vi "SetAtributes.vi"() -> ()   [LabVIEW 2012]
uses:
  <vilib>/Instr/_visa.llb/VISA Configure Serial Port (Instr).vi
panel:
  out "Coef start vasak":string
  out "Coef start parem":string
  in  "Vasak":bool
  out "Konstant vasak":dbl format="%#_4g"
  in  "Raskus vasak":dbl=200.0
  out "Coef OUT vasak":string
  out "Coef IN vasak":string
  in  "Parem":bool
  out "Coef IN parem":string
  out "Coef OUT parem":string
  out "Konstant parem":dbl format="%#_4g"
  in  "Raskus parem":dbl=200.0
  out "parem":dbl
  out "vasak":dbl
  in  "Mitu väärtust":i32=100
  in  "Kalibreeri":bool
  out "Pausi (oote) perioodi vaste":string
  in  "Pausi (oote) periood":string
  out "Salvestusperioodi vaste":string
  in  "Salvestusperiood":string
  out "Max vaste":string
  in  "Max":string
  in  "Pausi (oote) periood":bool
  in  "Salvestusperiood":bool
  in  "Max lävend":bool
  out "Aja vaste":string
  out "Min vaste":string
  in  "Min":string
  in  "Säti min lävend":bool
  in  "stop":bool
  in  "Säti aeg":bool
  in  "Kell":string
  in  "Kuupäev":string
  out "string 4":string
  in  "VISA Refnum in":refnum<visa-resource-name>="COM1"
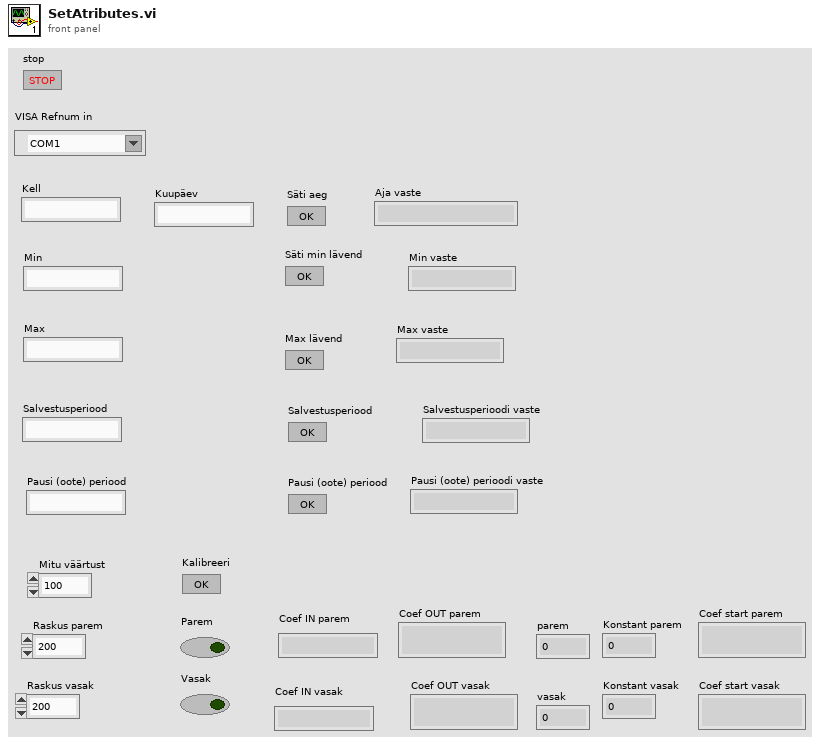
[diagram p1: front panel]
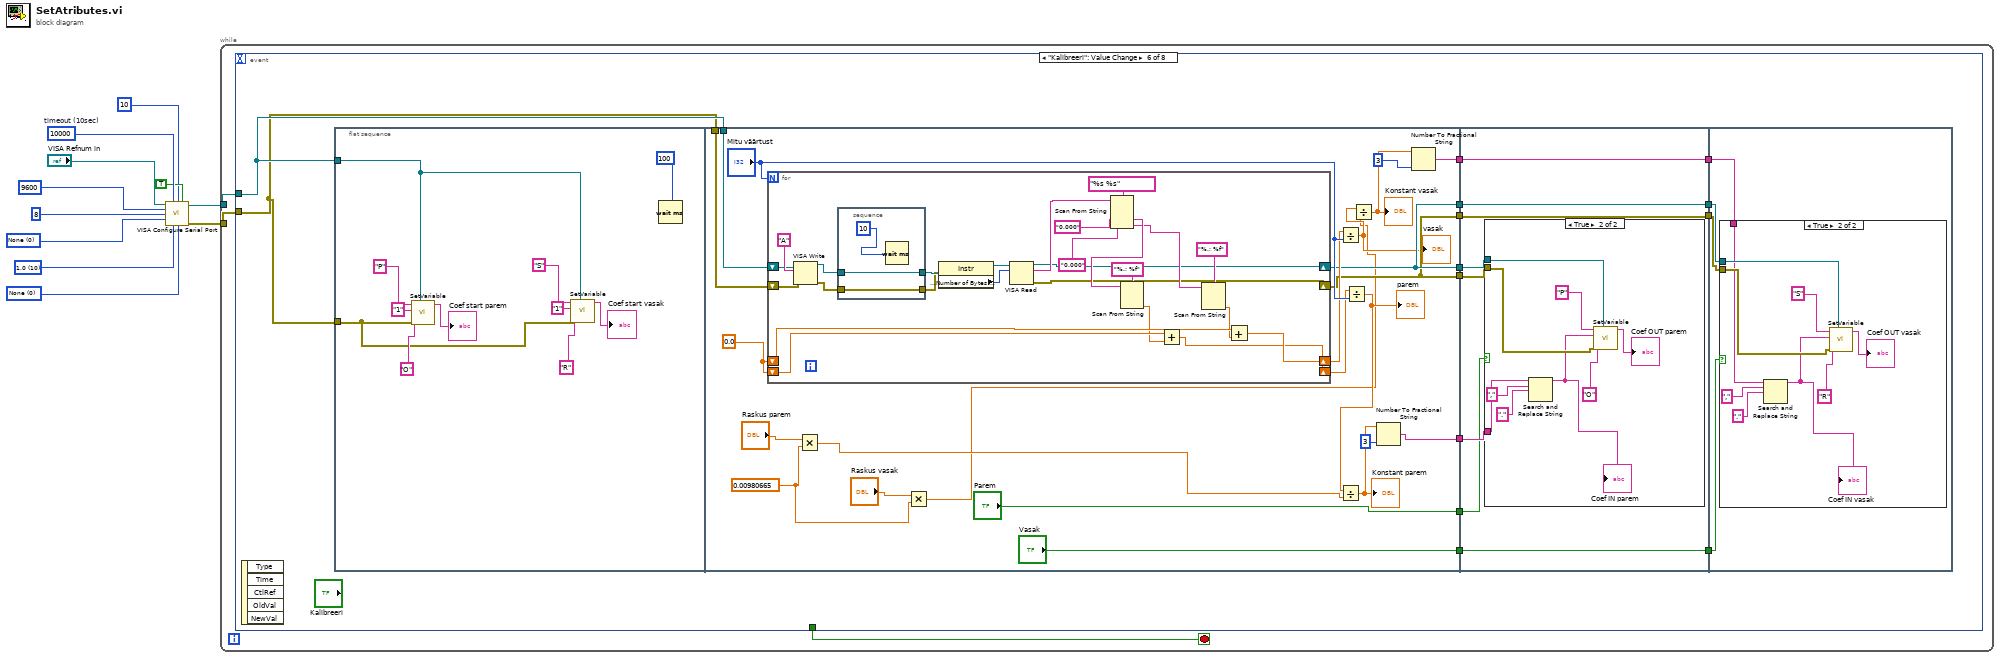
[diagram p0: block diagram]
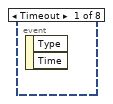
[diagram p2: hidden frame]
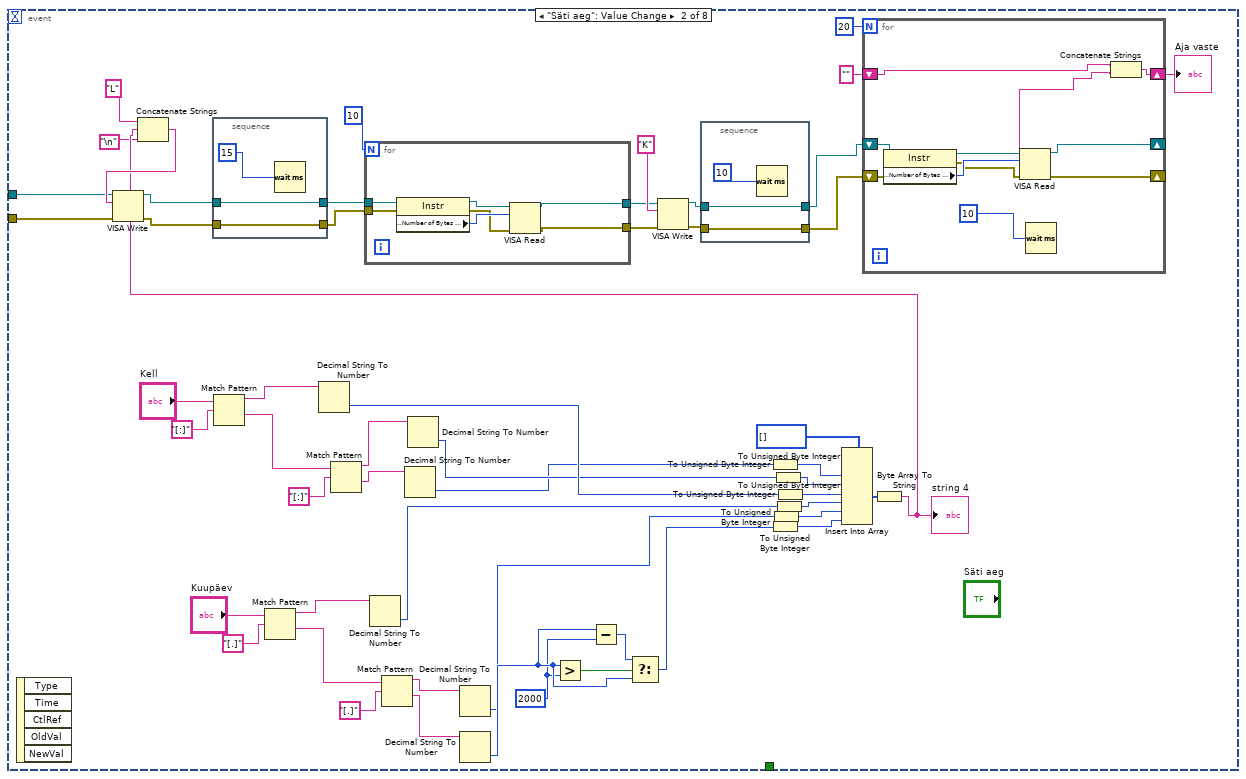
[diagram p3: hidden frame]
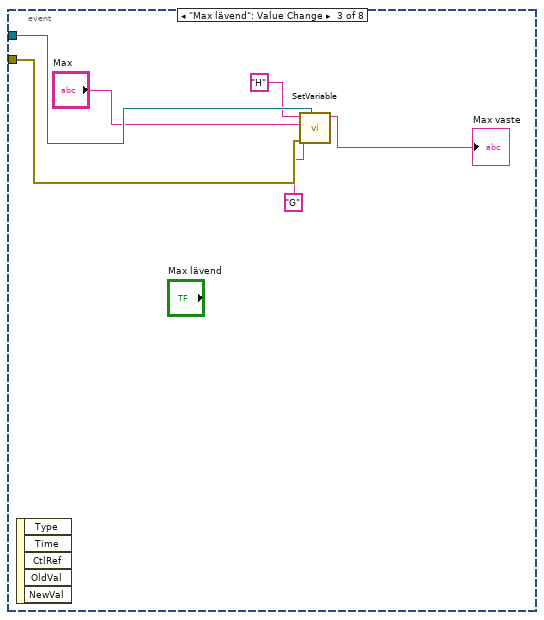
[diagram p4: hidden frame]
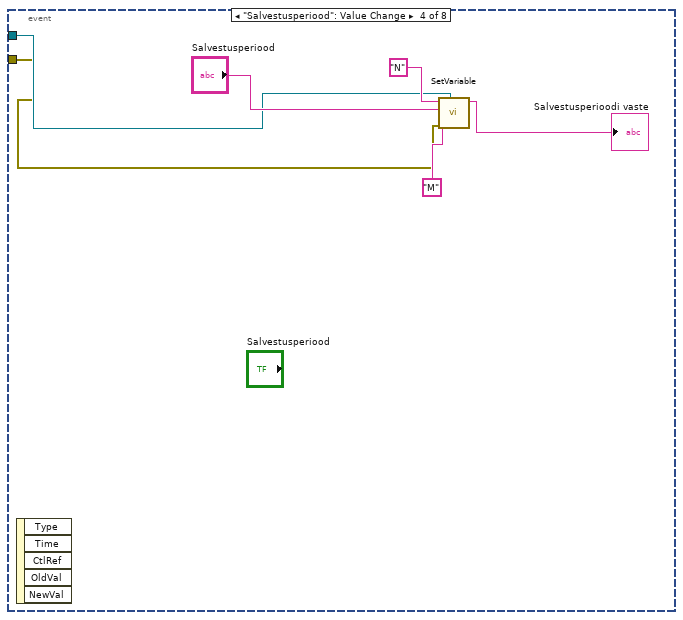
[diagram p5: hidden frame]
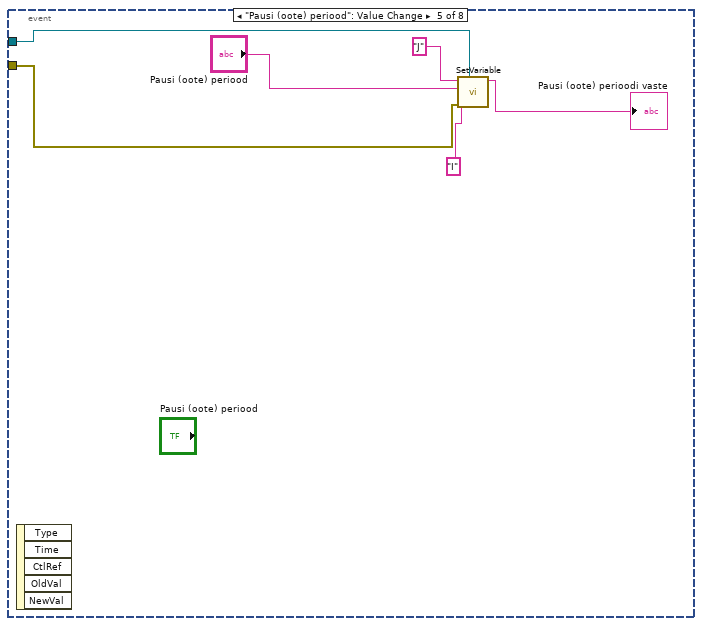
[diagram p6: hidden frame]
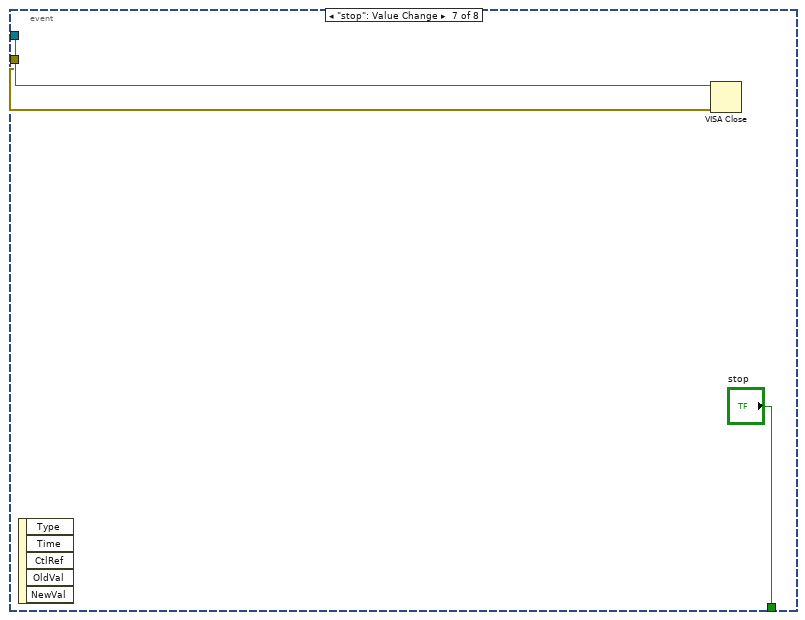
[diagram p9: hidden frame]
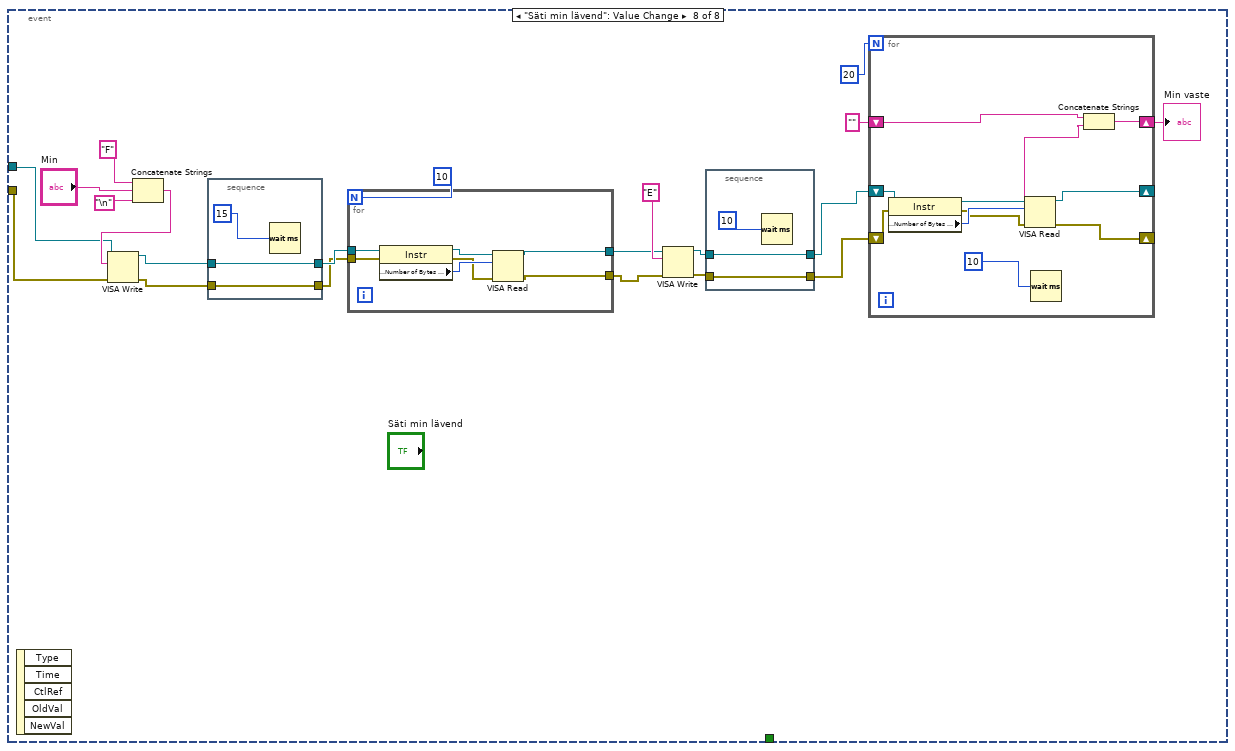
[diagram p10: hidden frame]
diagram:
  w11 = u16 0 items=["None"=0, "XON/XOFF"=1, "RTS/CTS"=2, "DTR/DSR"=4] ("flow control")
  w10 = u16 10 items=["1.0"=10, "1.5"=15, "2.0"=20] ("stop bits")
  w9 = u16 0 items=["None", "Odd", "Even", "Mark", "Space"] ("parity")
  w5 = u32 10000  # timeout (10sec)
  n1 = call-poly "VISA Configure Serial Port"("VISA resource name"="VISA Refnum in", "timeout (10sec)"=w5, "termination char\n(0xA = '\\n' = LF)"=u8 10 ("termination char\n(0xA = '\\n' = LF)"), "Enable Termination\nChar (T)"=TRUE ("Enable Termination\nChar (T)"), "baud rate (9600)"=u32 9600 ("baud rate"), "data bits (8)"=u16 8 ("data bits"), "parity (0:none)"=w9, "stop bits (10: 1 bit)"=w10, "flow control (0:none)"=w11) -> ("VISA resource name out"=w2:refnum<visa-resource-name>, "error out"=w1:errorcluster)  [unwired: 1 in, 4 out]
  n2 = while {
    tunnel: w2 -> [w14]
    tunnel: w1 -> [w13]
    stop <- w12 stop-if-true
    n3 = event shown="[5] \"Kalibreeri\": Value Change" {
      selector: _ -> [_ _ _ _ _ _ _ _]
      dyn-events: _ -> [_ _ _ _ _ _ _ _]
      timeout: _ -> [_ _ _ _ _ _ _ _]
      tunnel: w14 -> [_ w18 w97 w99 w104 w111 w217 w226]
      tunnel: w13 -> [_ w17 w96 w98 w105 w110 w216 w227]
      tunnel: [_ _ _ _ _ _ "stop" _] -> w12
      event Timeout {
        n4 = event-data() -> ()  [unwired: 1 in, 2 out]
      }
      event "Säti aeg": Value Change {
        w32 = 2000 ("y")
        n5 = event-data() -> ()  [unwired: 1 in, 5 out]
        n6 = Match Pattern(string="Kell", regular expression="[:]" ("search string/char (-)")) -> (before substring=w24:string, after substring=w25:string)  [unwired: 1 in, 2 out]
        n7 = Match Pattern(string="Kuupäev", regular expression="[.]" ("search string/char (-)")) -> (before substring=w38:string, after substring=w39:string)  [unwired: 1 in, 2 out]
        n8 = Decimal String To Number(string=w24) -> (number=w21:i32)  [unwired: 2 in, 1 out]
        n9 = Match Pattern(string=w25, regular expression="[:]" ("search string/char (-)")) -> (before substring=w23:string, after substring=w22:string)  [unwired: 1 in, 2 out]
        n10 = Decimal String To Number(string=w38) -> (number=w29:i32)  [unwired: 2 in, 1 out]
        n11 = Match Pattern(string=w39, regular expression="[.]" ("search string/char (-)")) -> (before substring=w37:string, after substring=w36:string)  [unwired: 1 in, 2 out]
        n12 = Decimal String To Number(string=w22) -> (number=w19:i32)  [unwired: 2 in, 1 out]
        n13 = Decimal String To Number(string=w23) -> (number=w20:i32)  [unwired: 2 in, 1 out]
        n14 = Decimal String To Number(string=w37) -> (number=w30:i32)  [unwired: 2 in, 1 out]
        n15 = Decimal String To Number(string=w36) -> (number=w33:i32)  [unwired: 2 in, 1 out]
        n16 = Greater?(x=w33, y=w32) -> (0:w35:bool)
        n17 = Subtract(x=w33, y=w32) -> (x-y=w34:i32)
        n18 = Select(t=w34, s=w35, f=w33) -> (s? t:f=w31:i32)
        n19 = To Unsigned Byte Integer(number=w19) -> (unsigned 8bit integer=w57:u8)
        n20 = To Unsigned Byte Integer(number=w31) -> (unsigned 8bit integer=w50:u8)
        n21 = To Unsigned Byte Integer(number=w30) -> (unsigned 8bit integer=w51:u8)
        n22 = To Unsigned Byte Integer(number=w20) -> (unsigned 8bit integer=w54:u8)
        n23 = To Unsigned Byte Integer(number=w29) -> (unsigned 8bit integer=w52:u8)
        n24 = To Unsigned Byte Integer(number=w21) -> (unsigned 8bit integer=w53:u8)
        n25 = Insert Into Array(array=u8[] [], new element #1=w57, new element #2=w54, new element #3=w53, new element #4=w52, new element #5=w51, new element #6=w50) -> (w56:u8[])  [unwired: 1 in]
        n26 = Byte Array To String(unsigned byte array=w56) -> (string=w55:string)
        "string 4" <- w55
        n27 = Concatenate Strings("L" ("Command String"), w55, "\n") -> (w59:string)
        n28 = VISA Write(VISA resource name=w18, write buffer=w59, error in (no error)=w17) -> (VISA resource name out=w64:refnum<visa-resource-name>, error out=w63:errorcluster)  [unwired: 1 out]
        n29 = stacked-sequence {
          tunnel: w63 -> [w91]
          tunnel: [w91] -> w61
          tunnel: w64 -> [w90]
          tunnel: [w90] -> w62
          frame #0 {
            n30 = Wait (ms)(milliseconds to wait=u32 15 ("delay Command")) -> ()  [unwired: 1 out]
          }
        }
        n31 = for {
          N: 10 -> [_]
          tunnel: w62 -> [w85]
          tunnel: w61 -> [w84]
          tunnel: [w80] -> w47
          tunnel: [w79] -> w46
          n32 = property class="Instr"(reference=w85, error in=w84) -> (reference out=w83:refnum<visa-resource-name>, error out=w81:errorcluster, "Serial Settings:Number of Bytes at Serial Port"=w82:u32)
          n33 = VISA Read(VISA resource name=w83, byte count=w82, error in (no error)=w81) -> (VISA resource name out=w80:refnum<visa-resource-name>, error out=w79:errorcluster)  [unwired: 2 out]
        }
        n34 = VISA Write(VISA resource name=w47, write buffer="K" ("File name string"), error in (no error)=w46) -> (VISA resource name out=w66:refnum<visa-resource-name>, error out=w65:errorcluster)  [unwired: 1 out]
        n35 = stacked-sequence {
          tunnel: w65 -> [w88]
          tunnel: [w88] -> w48
          tunnel: w66 -> [w87]
          tunnel: [w87] -> w49
          frame #0 {
            n36 = Wait (ms)(milliseconds to wait=u32 10 ("delay Input")) -> ()  [unwired: 1 out]
          }
        }
        n37 = for {
          N: 20 -> [_]
          shift-right: [w70] -> w15
          shift-left: "" -> [w69]
          shift-right: [w76] -> _
          shift-left: w49 -> [w74]
          shift-right: [w73] -> _
          shift-left: w48 -> [w72]
          n38 = property class="Instr"(reference=w74, error in=w72) -> (reference out=w78:refnum<visa-resource-name>, error out=w75:errorcluster, "Serial Settings:Number of Bytes at Serial Port"=w77:u32)
          n39 = VISA Read(VISA resource name=w78, byte count=w77, error in (no error)=w75) -> (VISA resource name out=w76:refnum<visa-resource-name>, read buffer=w68:string, error out=w73:errorcluster)  [unwired: 1 out]
          n40 = Wait (ms)(milliseconds to wait=u32 10 ("delay Input 2")) -> ()  [unwired: 1 out]
          n41 = Concatenate Strings(w69, w68) -> (w70:string)
        }
        "Aja vaste" <- w15
      }
      event "Max lävend": Value Change {
        n42 = event-data() -> ()  [unwired: 1 in, 5 out]
        n43 = call "SetVariable.vi"("VISA resource name"=w97, "error in (no error)"=w96, "Vaste käsk"="G", "Sisu"="Max", "Käsk"="H") -> ("Väljund"=→"Max vaste":string)  [unwired: 6 in]
      }
      event "Salvestusperiood": Value Change {
        n44 = event-data() -> ()  [unwired: 1 in, 5 out]
        n45 = call "SetVariable.vi"("VISA resource name"=w99, "error in (no error)"=w98, "Vaste käsk"="M", "Sisu"="Salvestusperiood", "Käsk"="N") -> ("Väljund"=→"Salvestusperioodi vaste":string)  [unwired: 6 in]
      }
      event "Pausi (oote) periood": Value Change {
        n46 = event-data() -> ()  [unwired: 1 in, 5 out]
        n47 = call "SetVariable.vi"("VISA resource name"=w104, "error in (no error)"=w105, "Vaste käsk"="I", "Sisu"="Pausi (oote) periood", "Käsk"="J") -> ("Väljund"=→"Pausi (oote) perioodi vaste":string)  [unwired: 6 in]
      }
      event "Kalibreeri": Value Change {
        n48 = event-data() -> ()  [unwired: 1 in, 5 out]
        n49 = flat-sequence {
          tunnel: w111 -> [w126]
          tunnel: w110 -> [w125]
          tunnel: w111 -> [w157]
          tunnel: w110 -> [w156]
          tunnel: [w144] -> w123
          tunnel: [w143] -> w122
          tunnel: [w148] -> w121
          tunnel: ["Parem"] -> w120
          tunnel: [w144] -> w118
          tunnel: [w143] -> w116
          tunnel: ["Vasak"] -> w114
          tunnel: [w136] -> w112
          tunnel: w123 -> [w193]
          tunnel: w122 -> [w192]
          tunnel: w121 -> [w191]
          tunnel: w120 -> [w190]
          tunnel: [w189] -> w119
          tunnel: w118 -> [w189]
          tunnel: [w188] -> w117
          tunnel: w116 -> [w188]
          tunnel: [w187] -> w115
          tunnel: w114 -> [w187]
          tunnel: [w186] -> w113
          tunnel: w112 -> [w186]
          tunnel: w119 -> [w206]
          tunnel: w117 -> [w205]
          tunnel: w115 -> [w204]
          tunnel: w113 -> [w203]
          frame #0 {
            n50 = call "SetVariable.vi"("VISA resource name"=w126, "error in (no error)"=w125, "Vaste käsk"="O", "Sisu"="1", "Käsk"="P") -> ("Väljund"=→"Coef start parem":string)  [unwired: 6 in]
            n51 = call "SetVariable.vi"("VISA resource name"=w126, "error in (no error)"=w125, "Vaste käsk"="R", "Sisu"="1", "Käsk"="S") -> ("Väljund"=→"Coef start vasak":string)  [unwired: 6 in]
            n52 = Wait (ms)(milliseconds to wait=u32 100) -> ()  [unwired: 1 out]
          }
          frame #1 {
            w135 = 0.00980665 ("y")
            w152 = 0.0 ("x")
            n53 = for {
              N: "Mitu väärtust" -> [_]
              shift-right: [w167] -> w144
              shift-left: w157 -> [w165]
              shift-right: [w166] -> w143
              shift-left: w156 -> [w164]
              shift-right: [w158] -> w153
              shift-left: w152 -> [w163]
              shift-right: [w159] -> w154
              shift-left: w152 -> [w162]
              n54 = VISA Write(VISA resource name=w165, write buffer="A" ("Command String"), error in (no error)=w164) -> (VISA resource name out=w181:refnum<visa-resource-name>, error out=w180:errorcluster)  [unwired: 1 out]
              n55 = stacked-sequence {
                tunnel: w180 -> [w185]
                tunnel: [w185] -> w176
                tunnel: w181 -> [w184]
                tunnel: [w184] -> w177
                frame #0 {
                  n56 = Wait (ms)(milliseconds to wait=u32 10 ("delay Command")) -> ()  [unwired: 1 out]
                }
              }
              n57 = property class="Instr"(reference=w177, error in=w176) -> (reference out=w179:refnum<visa-resource-name>, "Serial Settings:Number of Bytes at Serial Port"=w178:u32)  [unwired: 1 out]
              n58 = VISA Read(VISA resource name=w179, byte count=w178) -> (VISA resource name out=w167:refnum<visa-resource-name>, read buffer=w175:string, error out=w166:errorcluster)  [unwired: 1 in, 1 out]
              n59 = Scan From String(format string="%s %s", input string=w175, default 1="0.000", default 2="0.000") -> (output 1=w169:string, output 2=w168:string)  [unwired: 2 in, 3 out]
              n60 = Scan From String(format string="%.; %f", input string=w169) -> (output 1=w161:dbl)  [unwired: 3 in, 3 out]
              n61 = Add(x=w163, y=w161) -> (x+y=w158:dbl)
              n62 = Scan From String(format string="%.; %f", input string=w168) -> (output 1=w160:dbl)  [unwired: 3 in, 3 out]
              n63 = Add(x=w162, y=w160) -> (x+y=w159:dbl)
            }
            n64 = Multiply(x="Raskus parem", y=w135) -> (x*y=w150:dbl)
            n65 = Multiply(x="Raskus vasak", y=w135) -> (x*y=w138:dbl)
            n66 = Divide(x=w154, y="Mitu väärtust") -> (x/y=w139:dbl)
            "vasak" <- w139
            n67 = Divide(x=w153, y="Mitu väärtust") -> (x/y=w149:dbl)
            "parem" <- w149
            n68 = Divide(x=w149, y=w150) -> (x/y=w147:dbl)
            "Konstant parem" <- w147
            n69 = Divide(x=w139, y=w138) -> (x/y=w141:dbl)
            "Konstant vasak" <- w141
            n70 = Number To Fractional String(number=w147, precision (6)=i16 3) -> (F-format string=w148:string)  [unwired: 2 in]
            n71 = Number To Fractional String(number=w141, precision (6)=i16 3) -> (F-format string=w136:string)  [unwired: 2 in]
          }
          frame #2 {
            n72 = case shown="True" w190 {
              tunnel: w193 -> [_ w199]
              tunnel: w192 -> [_ w198]
              tunnel: w191 -> [_ w197]
              frame False {
              }
              frame True {
                n73 = Search and Replace String(input string=w197, search string=",", replace string="." ("replace string (\"\")")) -> (result string=w194:string)  [unwired: 5 in, 3 out]
                "Coef IN parem" <- w194
                n74 = call "SetVariable.vi"("VISA resource name"=w199, "error in (no error)"=w198, "Vaste käsk"="O", "Sisu"=w194, "Käsk"="P") -> ("Väljund"=→"Coef OUT parem":string)  [unwired: 6 in]
              }
            }
          }
          frame #3 {
            n75 = case shown="True" w204 {
              tunnel: w206 -> [_ w212]
              tunnel: w205 -> [_ w211]
              tunnel: w203 -> [_ w207]
              frame False {
              }
              frame True {
                n76 = Search and Replace String(input string=w207, search string=",", replace string="." ("replace string (\"\")")) -> (result string=w208:string)  [unwired: 5 in, 3 out]
                "Coef IN vasak" <- w208
                n77 = call "SetVariable.vi"("VISA resource name"=w212, "error in (no error)"=w211, "Vaste käsk"="R", "Sisu"=w208, "Käsk"="S") -> ("Väljund"=→"Coef OUT vasak":string)  [unwired: 6 in]
              }
            }
          }
        }
      }
      event "stop": Value Change {
        n78 = event-data() -> ()  [unwired: 1 in, 5 out]
        n79 = VISA Close(VISA resource name=w217, error in (no error)=w216) -> ()  [unwired: 1 out]
      }
      event "Säti min lävend": Value Change {
        n80 = event-data() -> ()  [unwired: 1 in, 5 out]
        n81 = Concatenate Strings("F" ("Command String"), "Min", "\n") -> (w234:string)
        n82 = VISA Write(VISA resource name=w226, write buffer=w234, error in (no error)=w227) -> (VISA resource name out=w239:refnum<visa-resource-name>, error out=w238:errorcluster)  [unwired: 1 out]
        n83 = stacked-sequence {
          tunnel: w238 -> [w263]
          tunnel: [w263] -> w236
          tunnel: w239 -> [w262]
          tunnel: [w262] -> w237
          frame #0 {
            n84 = Wait (ms)(milliseconds to wait=u32 15 ("delay Command")) -> ()  [unwired: 1 out]
          }
        }
        n85 = for {
          N: 10 -> [_]
          tunnel: w237 -> [w260]
          tunnel: w236 -> [w259]
          tunnel: [w255] -> w225
          tunnel: [w254] -> w224
          n86 = property class="Instr"(reference=w260, error in=w259) -> (reference out=w258:refnum<visa-resource-name>, error out=w256:errorcluster, "Serial Settings:Number of Bytes at Serial Port"=w257:u32)
          n87 = VISA Read(VISA resource name=w258, byte count=w257, error in (no error)=w256) -> (VISA resource name out=w255:refnum<visa-resource-name>, error out=w254:errorcluster)  [unwired: 2 out]
        }
        n88 = VISA Write(VISA resource name=w225, write buffer="E" ("File name string"), error in (no error)=w224) -> (VISA resource name out=w229:refnum<visa-resource-name>, error out=w228:errorcluster)  [unwired: 1 out]
        n89 = stacked-sequence {
          tunnel: w228 -> [w253]
          tunnel: [w253] -> w223
          tunnel: w229 -> [w252]
          tunnel: [w252] -> w222
          frame #0 {
            n90 = Wait (ms)(milliseconds to wait=u32 10 ("delay Input")) -> ()  [unwired: 1 out]
          }
        }
        n91 = for {
          N: 20 -> [_]
          shift-right: [w240] -> w219
          shift-left: "" -> [w241]
          shift-right: [w245] -> _
          shift-left: w222 -> [w243]
          shift-right: [w244] -> _
          shift-left: w223 -> [w246]
          n92 = property class="Instr"(reference=w243, error in=w246) -> (reference out=w250:refnum<visa-resource-name>, error out=w248:errorcluster, "Serial Settings:Number of Bytes at Serial Port"=w249:u32)
          n93 = VISA Read(VISA resource name=w250, byte count=w249, error in (no error)=w248) -> (VISA resource name out=w245:refnum<visa-resource-name>, read buffer=w242:string, error out=w244:errorcluster)  [unwired: 1 out]
          n94 = Wait (ms)(milliseconds to wait=u32 10 ("delay Input 2")) -> ()  [unwired: 1 out]
          n95 = Concatenate Strings(w241, w242) -> (w240:string)
        }
        "Min vaste" <- w219
      }
    }
  }
